vi "WritemmWaveMoving.vi"(8 "error in (no error)":errorcluster, 9 "Axis Moving = True":bool, 10 "mmWave Axis Name":string, 11 "UI MotionStatus in":refnum<class "UI MotionStatus.lvclass">) -> (0 "error out":errorcluster, 3 "UI MotionStatus out":refnum<class "UI MotionStatus.lvclass">)   [LabVIEW 2019, in "UI MotionStatus.lvclass"]
doc: "Use mmWave axis name to find numeric indicator refnum.\nwrite value."
uses:
  UI MotionStatus.lvclass
  UI MotionStatus.lvclass/UI MotionStatus.ctl
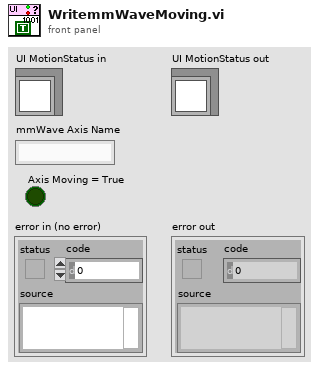
[diagram p1: front panel]
types:
  T1 = typedef "MotionStatusLEDCtrlRefs.ctl" = cluster{"BS1":refnum<vi>, "BS2":refnum<vi>, "BS3":refnum<vi>, "BS4":refnum<vi>, "RT1":refnum<vi>, "RT2":refnum<vi>, "RT3":refnum<vi>}
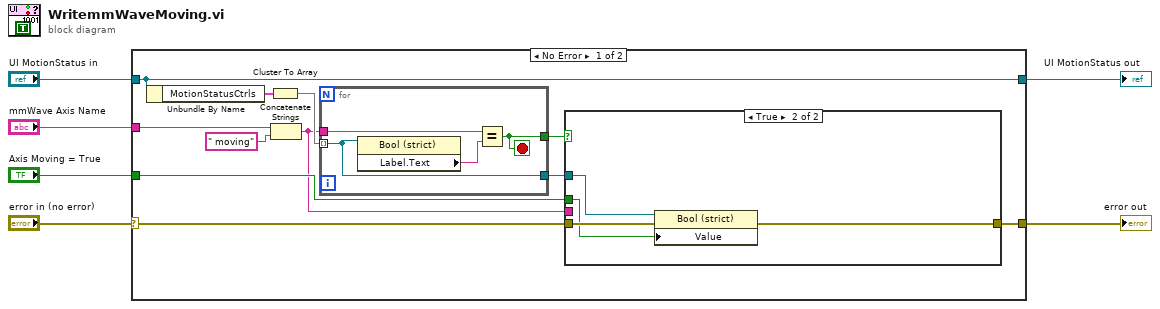
[diagram p0: block diagram]
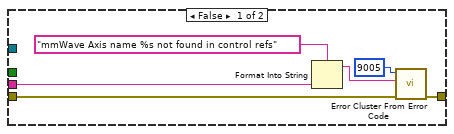
[diagram p2: hidden frame]
diagram:
  n1 = case shown="No Error" "error in (no error)" {
    selector: "error in (no error)" -> [w14 w33]
    tunnel: [w13 w33] -> w5
    tunnel: [w17 w32] -> w3
    tunnel: "UI MotionStatus in" -> [w17 w32]
    tunnel: "mmWave Axis Name" -> [w8 _]
    tunnel: "Axis Moving = True" -> [w10 _]
    frame No Error {
      n2 = Unbundle By Name(w17) -> ("MotionStatusCtrls"=w16:T1)
      n3 = Cluster To Array(cluster=w16) -> (array=w15:refnum<vi>[])
      n4 = Concatenate Strings(w8, " moving" ("string")) -> (w7:string)
      n5 = for {
        tunnel: w7 -> [w30]
        tunnel: w15 -> [w29] mode=indexing
        tunnel: [w29] -> w11
        tunnel: [w28] -> w12
        stop <- w28 stop-if-true
        n6 = property class="Bool (strict)"(reference=w29) -> ("Label.Text"=w31:string)  [unwired: 1 in, 2 out]
        n7 = Equal?(x=w30, y=w31) -> (x = y?=w28:bool)
      }
      n8 = case shown="True" w12 {
        tunnel: w7 -> [w20 _]
        tunnel: w14 -> [w19 w26]
        tunnel: [w18 w25] -> w13
        tunnel: w11 -> [_ w27]
        tunnel: w10 -> [_ w24]
        frame False {
          n9 = Format Into String(format string="mmWave Axis name %s not found in control refs", w20) -> (resulting string=w21:string)  [unwired: 2 in, 1 out]
          n10 = call <vilib>:"Error Cluster From Error Code.vi"("error in (no error)"=w19, "error message (\"\")"=w21, "error code (0)"=9005) -> ("error out"=w18:errorcluster)  [unwired: 6 in]
        }
        frame True {
          n11 = property class="Bool (strict)"(reference=w27, error in=w26, "Value"=w24) -> (error out=w25:errorcluster)  [unwired: 1 out]
        }
      }
    }
    frame Error {
    }
  }
  "error out" <- w5
  "UI MotionStatus out" <- w3
